vi "LineCutGateSweep.vi"(8 "Basename":string) -> ()   [LabVIEW 2021]
uses:
  <userlib>/Nanonis Prog Interface V5/Nanonis Prog Interface.lvlib
panel:
  out "Point Distance (nm)":dbl
  out "Total Distance (nm)":dbl
  in  "Increment Gate (V)":dbl=1.0
  in  "End Gate (V)":dbl=60.0
  in  "Start Gate (V)":dbl=-60.0
  in  "milliseconds\nbetween spectra":u32=500
  in  "Points":i32=200
  in  "End Y (m)":dbl format="%#_6p"
  in  "End X (m)":dbl format="%#_6p"
  in  "Start Y (m)":dbl format="%#_6p"
  in  "Start X (m)":dbl format="%#_6p"
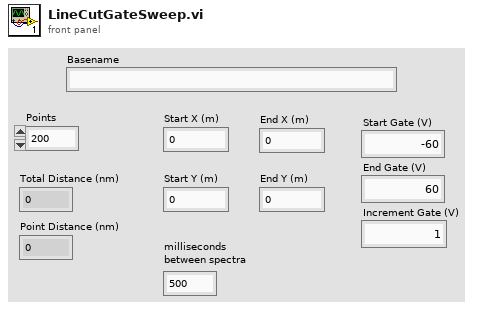
[diagram p1: front panel]
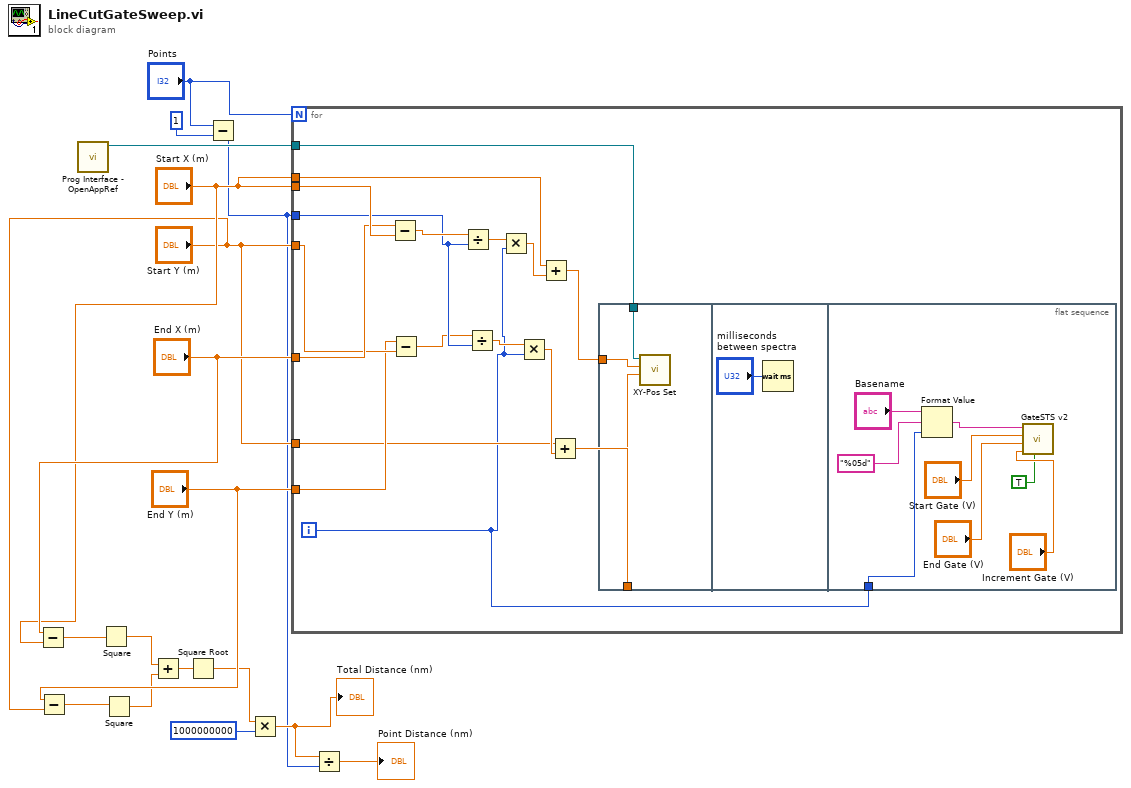
[diagram p0: block diagram]
diagram:
  n1 = Subtract(x="End X (m)", y="Start X (m)") -> (x-y=w12:dbl)
  n2 = Subtract(x="End Y (m)", y="Start Y (m)") -> (x-y=w9:dbl)
  n3 = call <userlib>:"Prog Interface - OpenAppRef.vi"() -> ("Application reference"=w17:refnum<vi>)  [unwired: 6 in, 1 out]
  n4 = Square(x=w12) -> (x^2=w7:dbl)
  n5 = Square(x=w9) -> (x^2=w6:dbl)
  n6 = Add(x=w7, y=w6) -> (x+y=w8:dbl)
  n7 = Square Root(x=w8) -> (sqrt(x)=w5:dbl)
  n8 = Subtract(x="Points", y=1) -> (x-y=w2:i32)
  n9 = Multiply(x=w5, y=1000000000) -> (x*y=w3:dbl)
  "Total Distance (nm)" <- w3
  n10 = for {
    N: "Points" -> [_]
    tunnel: "Start X (m)" -> [w34]
    tunnel: "End X (m)" -> [w33]
    tunnel: "Start Y (m)" -> [w32]
    tunnel: "End Y (m)" -> [w31]
    tunnel: w2 -> [w29]
    tunnel: w17 -> [w27]
    tunnel: "Start X (m)" -> [w25]
    tunnel: "Start Y (m)" -> [w22]
    i -> [w19]
    n11 = Subtract(x=w33, y=w34) -> (x-y=w30:dbl)
    n12 = Subtract(x=w31, y=w32) -> (x-y=w28:dbl)
    n13 = Divide(x=w30, y=w29) -> (x/y=w18:dbl)
    n14 = Divide(x=w28, y=w29) -> (x/y=w26:dbl)
    n15 = Multiply(x=w18, y=w19) -> (x*y=w24:dbl)
    n16 = Multiply(x=w26, y=w19) -> (x*y=w23:dbl)
    n17 = Add(x=w25, y=w24) -> (x+y=w20:dbl)
    n18 = Add(x=w22, y=w23) -> (x+y=w21:dbl)
    n19 = flat-sequence {
      tunnel: w27 -> [w37]
      tunnel: w21 -> [w36]
      tunnel: w20 -> [w35]
      tunnel: w19 -> [w42]
      frame #0 {
        n20 = call <userlib>:"XY-Pos Set.vi"("Y (m)"=w36, "X (m)"=w35, "Application ref in"=w37) -> ()  [unwired: 5 in, 2 out]
      }
      frame #1 {
        n21 = Wait (ms)(milliseconds to wait="milliseconds\nbetween spectra") -> ()  [unwired: 1 out]
      }
      frame #2 {
        n22 = Format Value(string ("")="Basename", format string="%05d", value (0)=w42) -> (output string=w39:string)
        n23 = call "GateSTS v2.vi"("Store\nSecond Gate?"=TRUE ("Store\nSecond Gate?"), "Increment Gate (V)"="Increment Gate (V)", "End Gate (V)"="End Gate (V)", "Start Gate (V)"="Start Gate (V)", "Basename"=w39) -> ()  [unwired: 5 in, 1 out]
      }
    }
  }
  n24 = Divide(x=w3, y=w2) -> (x/y=→"Point Distance (nm)":dbl)
